vi "Create Table.vi"(0 "PDF Report IN":refnum<class "PDF Report Class.lvclass">=refnum, 1 "Repeat Headers Column":bool=TRUE, 2 "Table columnWidth [ ]":sgl[](array[numeric]), 5 "Column Headers 2D [ ]":string[][](array[string]), 7 "Row Headers 1D [ ]":string[](array[string]), 9 "Text Data 2D [ ]":string[][](array[string]), 11 "error in (no error)":errorcluster, 12 "Image to Add [ ]":T1 {"Scale" format="%#_g %"}) -> (4 "PDF Report duplicate":refnum<class "PDF Report Class.lvclass">, 8 "PDF Table":refnum<class "Pdfp Table Class.lvclass">, 15 "error out":errorcluster)   [LabVIEW 2019, in "Exaprom PDF.lvlib"]
doc: "Version 2.0\nDeveloped by Jean-Marc Simard\nCopyright © 2012, Exaprom Inc.\nAll rights reserved.\nLicense: BSD\n\nWith iTextSharp 4.1.6 (http://itextsharp.sourceforge.net)\nunder Mozilla Public License Version 1.1\n(http://www.mozilla.org/MPL/MPL-1.1.html)"
uses:
  LV Class/PDF Report Class/PDF Report Class.lvclass
  LV Class/Fonts Class/Font Class.lvclass
  LV Class/Header and Footer Class/Header and Footer Class.lvclass
  Controls/General Controls/Image to Add [ ].ctl
  Controls/Image Controls/Image Scale.ctl
  LV Class/Pdfp Table Class/Pdfp Table Class.lvclass
  Controls/Table Controls/Table type.ctl
  Exaprom PDF.lvlib
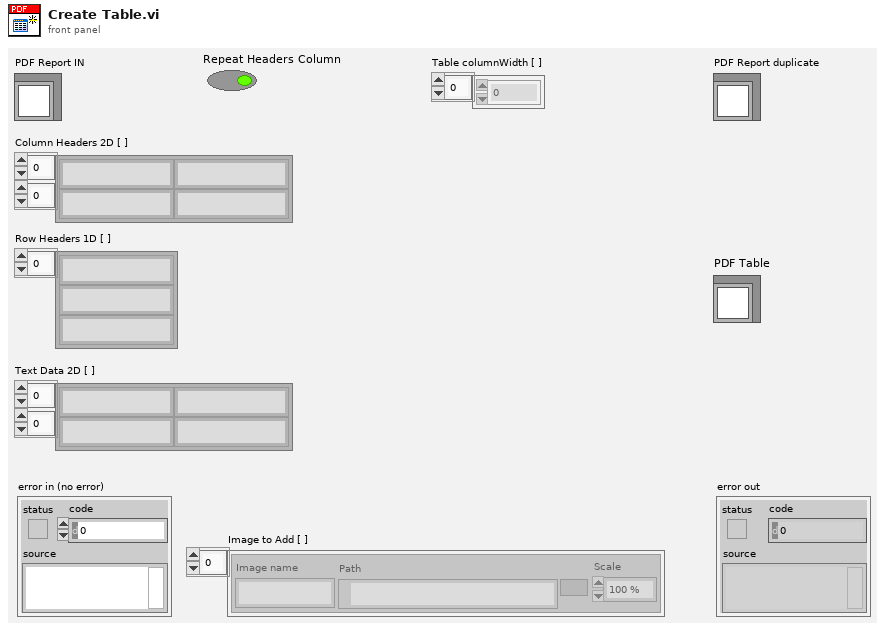
[diagram p1: front panel]
types:
  T1 = typedef "Exaprom PDF.lvlib/Image to Add [ ].ctl" = cluster{"Image name":string, "Path":path, "Scale":T2}[]
  T2 = typedef "Exaprom PDF.lvlib/Image Scale.ctl" = sgl
  T3 = typedef "Exaprom PDF.lvlib/Table type.ctl" = enum16{"Standard", "Customized"}
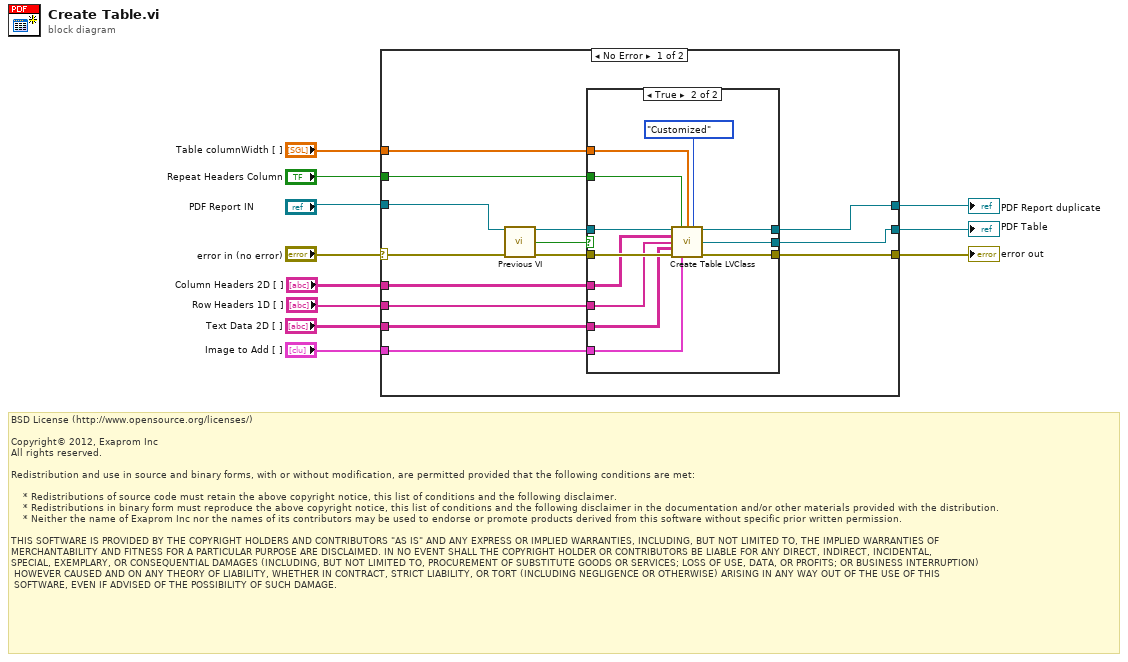
[diagram p0: block diagram]
diagram:
  # "BSD License (http://www.opensource.org/licenses/)\n\nCopyright© 2012, Exaprom Inc\nAll rights reserved.\n\nRedistribution and use in source and binary forms, with or without modification, are permitted provided that the following conditions are met:\n\n    * Redistributions of source code must retain the above copyright notice, this list of conditions and the following disclaimer.\n    * Redistributions in binary form must reproduce the above copyright notice, this list of conditions and the following disclaimer in the documentation and/or other materials provided with the distribution.\n    * Neither the name of Exaprom Inc nor the names of its contributors may be used to endorse or promote products derived from this software without specific prior written permission.\n\nTHIS SOFTWARE IS PROVIDED BY THE COPYRIGHT HOLDERS AND CONTRIBUTORS \"AS IS\" AND ANY EXPRESS OR IMPLIED WARRANTIES, INCLUDING, BUT NOT LIMITED TO, THE IMPLIED WARRANTIES OF \nMERCHANTABILITY AND FITNESS FOR A PARTICULAR PURPOSE ARE DISCLAIMED. IN NO EVENT SHALL THE COPYRIGHT HOLDER OR CONTRIBUTORS BE LIABLE FOR ANY DIRECT, INDIRECT, INCIDENTAL,\nSPECIAL, EXEMPLARY, OR CONSEQUENTIAL DAMAGES (INCLUDING, BUT NOT LIMITED TO, PROCUREMENT OF SUBSTITUTE GOODS OR SERVICES; LOSS OF USE, DATA, OR PROFITS; OR BUSINESS INTERRUPTION)\n HOWEVER CAUSED AND ON ANY THEORY OF LIABILITY, WHETHER IN CONTRACT, STRICT LIABILITY, OR TORT (INCLUDING NEGLIGENCE OR OTHERWISE) ARISING IN ANY WAY OUT OF THE USE OF THIS\n SOFTWARE, EVEN IF ADVISED OF THE POSSIBILITY OF SUCH DAMAGE."
  n1 = case shown="No Error" "error in (no error)" {
    selector: "error in (no error)" -> [w21 w41]
    tunnel: "PDF Report IN" -> [w19 w40]
    tunnel: [w15 w40] -> w10
    tunnel: [w25 w41] -> w5
    tunnel: "Table columnWidth [ ]" -> [w22 _]
    tunnel: [w24 _] -> w1
    tunnel: "Repeat Headers Column" -> [w23 _]
    tunnel: "Image to Add [ ]" -> [w17 _]
    tunnel: "Column Headers 2D [ ]" -> [w14 _]
    tunnel: "Row Headers 1D [ ]" -> [w13 _]
    tunnel: "Text Data 2D [ ]" -> [w12 _]
    frame No Error {
      n2 = call "Previous VI.vi"("PDF Report IN"=w19, "error in (no error)"=w21) -> ("PDF Report OUT"=w16:refnum<class "PDF Report Class.lvclass">, "Execute Actual VI"=w18:bool, "error out"=w20:errorcluster)  [unwired: 11 out]
      n3 = case shown="True" w18 {
        tunnel: [w27 w39] -> w25
        tunnel: [_ w38] -> w24
        tunnel: w23 -> [_ w30]
        tunnel: w22 -> [_ w29]
        tunnel: w20 -> [w27 w37]
        tunnel: w17 -> [_ w36]
        tunnel: w16 -> [w26 w35]
        tunnel: [w26 w34] -> w15
        tunnel: w14 -> [_ w33]
        tunnel: w13 -> [_ w32]
        tunnel: w12 -> [_ w31]
        frame False {
        }
        frame True {
          n4 = call "Create Table LVClass.vi"("PDF Report"=w35, "Repeat Headers Row"=w30, "Table columnWidth [ ]"=w29, "Table type"=Table_type."Customized", "Column Headers 2D [ ]"=w33, "Row Headers 1D [ ]"=w32, "Text Data 2D [ ]"=w31, "error in (no error)"=w37, "Image to Add [ ]"=w36) -> ("PDF Report duplicate"=w34:refnum<class "PDF Report Class.lvclass">, "PDF Table"=w38:refnum<class "Pdfp Table Class.lvclass">, "error out"=w39:errorcluster)  [unwired: 4 in]
        }
      }
    }
    frame Error {
    }
  }
  "PDF Report duplicate" <- w10
  "PDF Table" <- w1
  "error out" <- w5
